vi "NanoScan Get Info.vi"(0 "VISA Ref":refnum<visa-resource-name>, 2 "Wait for Reply (T)":bool=TRUE, 11 "Error In":errorcluster) -> (4 "VISA Ref Dup":refnum<visa-resource-name>, 8 "Reply":string, 13 "Connected":bool, 15 "Error Out":errorcluster)   [LabVIEW 2020]
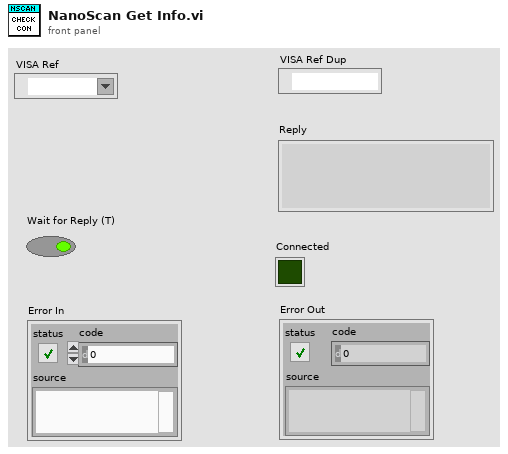
[diagram p1: front panel]
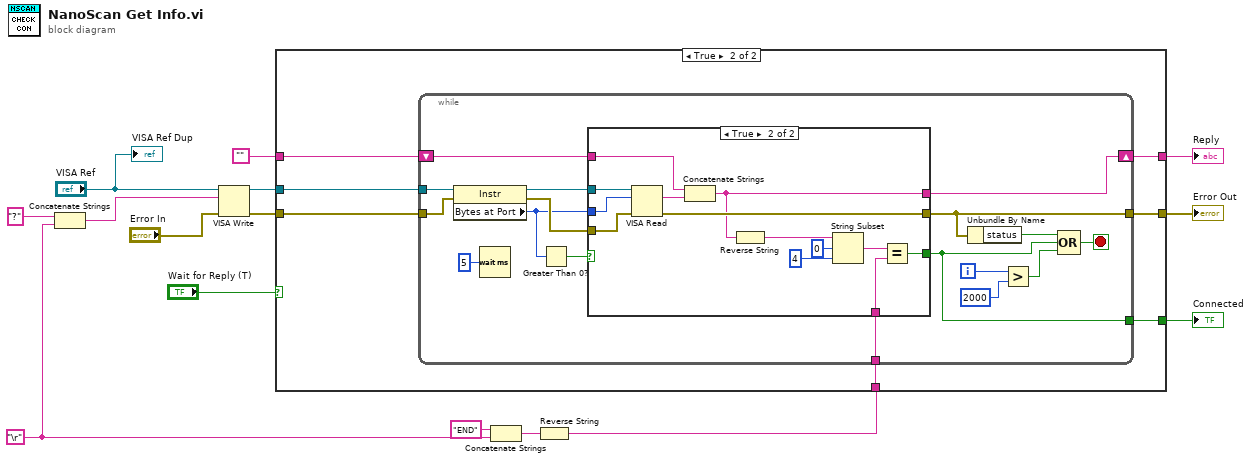
[diagram p0: block diagram]
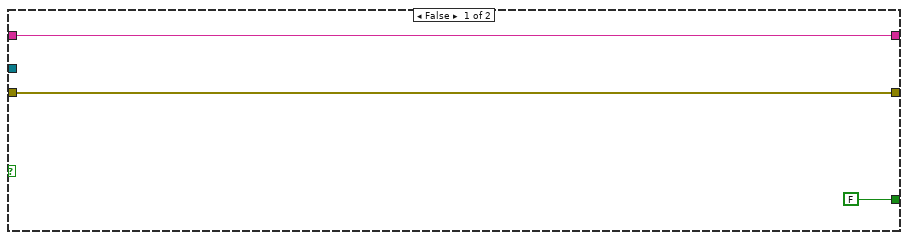
[diagram p2: hidden frame]
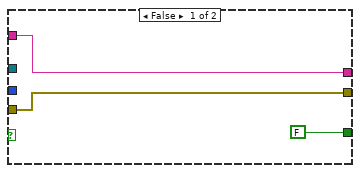
[diagram p3: hidden frame]
diagram:
  w5 = "\r"
  n1 = Concatenate Strings("?" ("Command"), w5) -> (w15:string)
  n2 = VISA Write(VISA resource name="VISA Ref", write buffer=w15, error in (no error)="Error In") -> (VISA resource name out=w14:refnum<visa-resource-name>, error out=w13:errorcluster)  [unwired: 1 out]
  n3 = Concatenate Strings("END" ("string"), w5) -> (w3:string)
  n4 = Reverse String(1:w3) -> (0:w2:string)
  n5 = case shown="True" "Wait for Reply (T)" {
    tunnel: w14 -> [_ w21]
    tunnel: w13 -> [w18 w20]
    tunnel: "" -> [w17 w25]
    tunnel: [w17 w24] -> w7
    tunnel: [w18 w23] -> w9
    tunnel: w2 -> [_ w22]
    tunnel: [FALSE w19] -> w6
    frame False {
    }
    frame True {
      n6 = while {
        tunnel: w21 -> [w42]
        tunnel: w20 -> [w41]
        shift-right: [w30] -> w24
        shift-left: w25 -> [w31]
        tunnel: [w28] -> w23
        tunnel: w22 -> [w27]
        tunnel: [w26] -> w19
        i -> [w40]
        stop <- w37 stop-if-true
        n7 = property class="Instr"(reference=w42, error in=w41) -> (reference out=w33:refnum<visa-resource-name>, error out=w34:errorcluster, "Bytes at Port"=w32:u32)
        n8 = Wait (ms)(milliseconds to wait=u32 5) -> ()  [unwired: 1 out]
        n9 = Greater Than 0?(x=w32) -> (x > 0?=w35:bool)
        n10 = case shown="True" w35 {
          tunnel: w34 -> [w45 w57]
          tunnel: w33 -> [_ w58]
          tunnel: w32 -> [_ w56]
          tunnel: w31 -> [w43 w55]
          tunnel: [w43 w52] -> w30
          tunnel: [w45 w53] -> w28
          tunnel: [FALSE w48] -> w26
          tunnel: w27 -> [_ w47]
          frame False {
          }
          frame True {
            n11 = VISA Read(VISA resource name=w58, byte count=w56, error in (no error)=w57) -> (read buffer=w54:string, error out=w53:errorcluster)  [unwired: 2 out]
            n12 = Concatenate Strings(w55, w54) -> (w52:string)
            n13 = Reverse String(1:w52) -> (0:w46:string)
            n14 = String Subset(string=w46, offset (0)=0, length (rest)=4 ("length (rest)")) -> (substring=w49:string)
            n15 = Equal?(x=w49, y=w47) -> (x = y?=w48:bool)
          }
        }
        n16 = Unbundle By Name(w28) -> ("status"=w29:bool)
        n17 = Greater?(x=w40, y=2000) -> (0:w38:bool)
        n18 = Compound Arithmetic op=OR(w29, w26, w38) -> (w37:bool)
      }
    }
  }
  "Reply" <- w7
  "Error Out" <- w9
  "Connected" <- w6
  "VISA Ref Dup" <- "VISA Ref"
